vi "Clear Interlock Alarm.vi"(8 "error in (no error)":errorcluster, 11 "2230G in":refnum<class "2230G.lvclass">) -> (0 "error out":errorcluster, 3 "2230G out":refnum<class "2230G.lvclass">)   [LabVIEW 2018, in "2230G.lvlib" / "2230G.lvclass"]
uses:
  2230G.lvclass
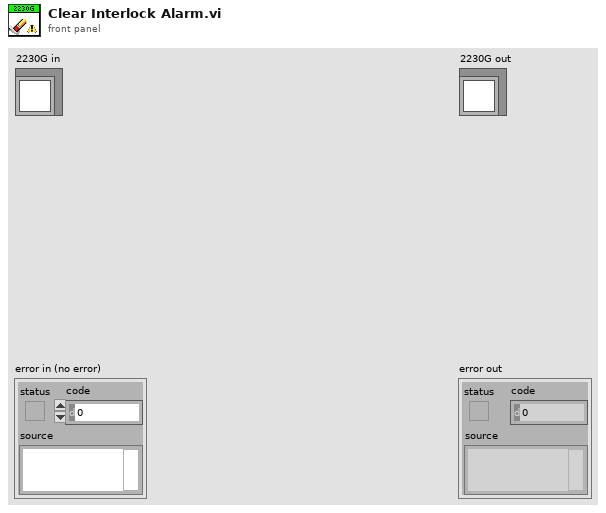
[diagram p1: front panel]
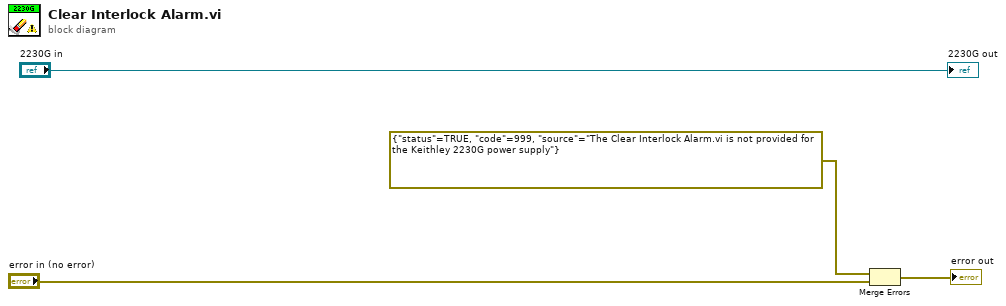
[diagram p0: block diagram]
diagram:
  n1 = Merge Errors(errorcluster {"status"=TRUE, "code"=999, "source"="The Clear Interlock Alarm.vi is not provided for the Keithley 2230G power supply"} ("error constant"), "error in (no error)") -> (→"error out":errorcluster)
  "2230G out" <- "2230G in"
